vi "Import from VASP DB.vi"(8 "error in (no error)":errorcluster) -> (0 "error out":errorcluster, 3 "All DFT Data Summary":T1)   [LabVIEW 2010]
uses:
  <vilib>/addons/database/Connection.llb/Conn ObjectReference.ctl
  <vilib>/addons/database/_DB Variant To Data/Database Variant To Data.xnode
  <vilib>/addons/database/Connection.llb/DB Tools Open Connec (Path).vi
  <vilib>/addons/database/Connection.llb/Conn Execute.vi
  <vilib>/addons/database/Recordset.llb/Rec Fetch Recordset Data (R).vi
  <vilib>/addons/database/Recordset.llb/Rec Destroy - Connection.vi
  <vilib>/addons/database/NI_Database_API.lvlib
panel:
  in  "Append to Last?":bool
  in  "Pre-Load Raw?":bool
  in  "UDL":path=path "D:/Ab-initio/VASP Calcs/VASP DB.udl"
  out "connection reference":T2
  in  "Cancel":bool
  in  "OK":bool
  in  "Search":bool
  in  "Query Build Cluster":T3={"Sample Check box"=TRUE, "Sample Comparison Type"="Contains", "Sample Name"="", "Logical Sample-Lot "="OR", "LotID Checkbox"=TRUE, "Lot Comparison Type"="Contains", "LotID Name"="", "Logical Lot-Date"="OR", "Date Checkbox"=TRUE, "Start Date"=timestamp(3375812149.928578 s since 1904-01-01), "End Date"=timestamp(3375812149.928578 s since 1904-01-01), "1st search column name"="Folder", "2nd search column name"="Pre_Structure"} {"Start Date" format="%<%X\n%x>T"; "End Date" format="%<%X\n%x>T"}
  in  "DFT Summary":i32(listbox)
  # "Get all results where"
  # "where"
  # "between these dates"
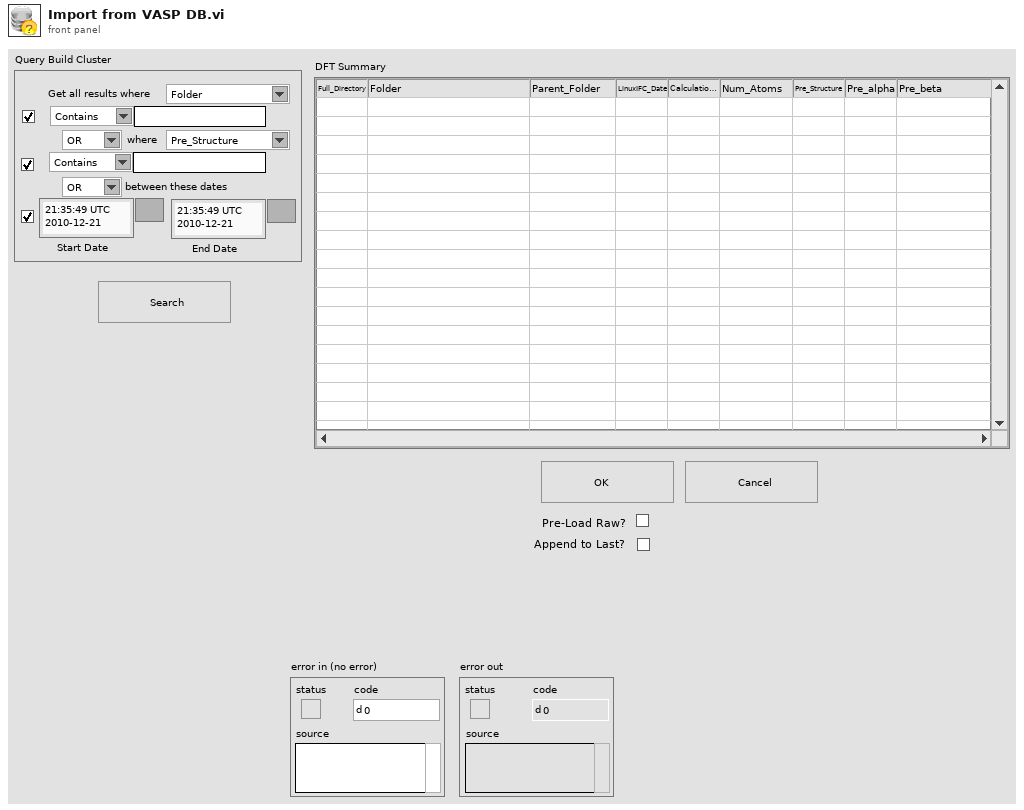
[diagram p1: front panel]
types:
  T1 = cluster{"Headers":string[], "Relaxation Data":string[][]}
  T2 = typedef "NI_Database_API.lvlib/Conn ObjectReference.ctl" = refnum<k1>
  T3 = cluster{"Sample Check box":bool, "Sample Comparison Type":string, "Sample Name":string, "Logical Sample-Lot ":string, "LotID Checkbox":bool, "Lot Comparison Type":string, "LotID Name":string, "Logical Lot-Date":string, "Date Checkbox":bool, "Start Date":timestamp, "End Date":timestamp, "1st search column name":string, "2nd search column name":string}
  T4 = typedef "NI_Database_API.lvlib/Rec ObjectReference.ctl" = refnum<k1>
  T5 = cluster{"ColHdrString":string[], "ItemNames":string[][]}
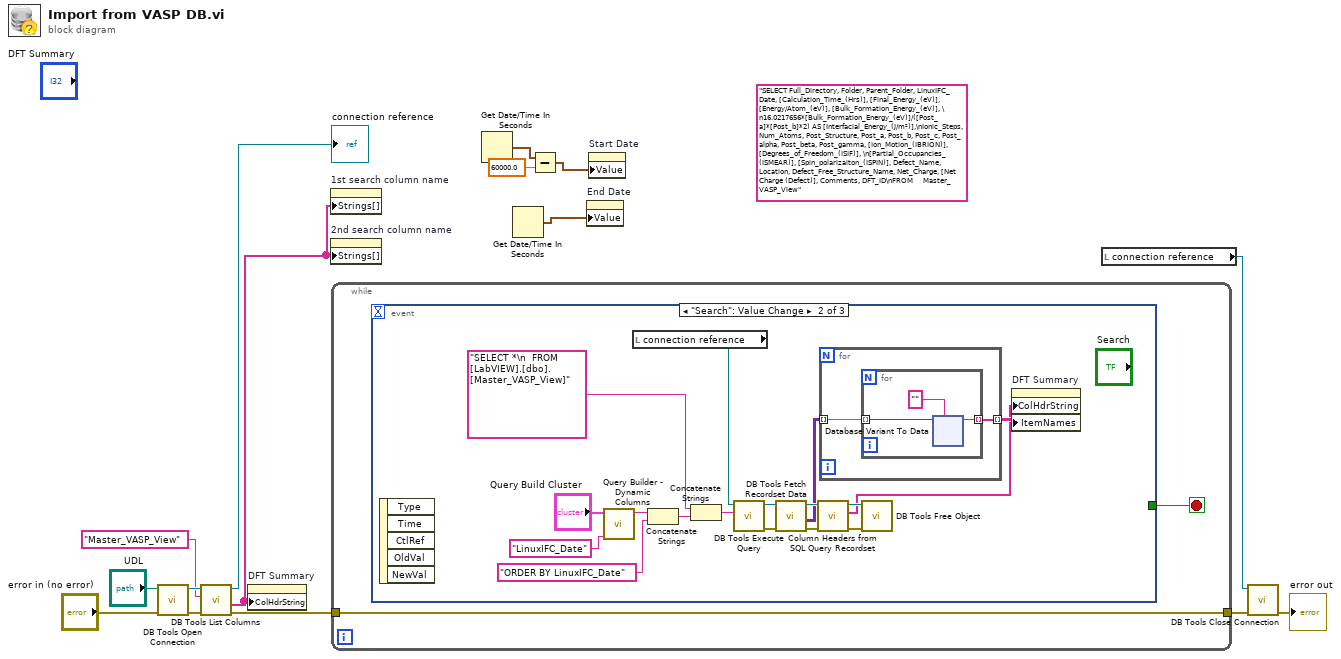
[diagram p0: block diagram]
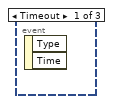
[diagram p2: hidden frame]
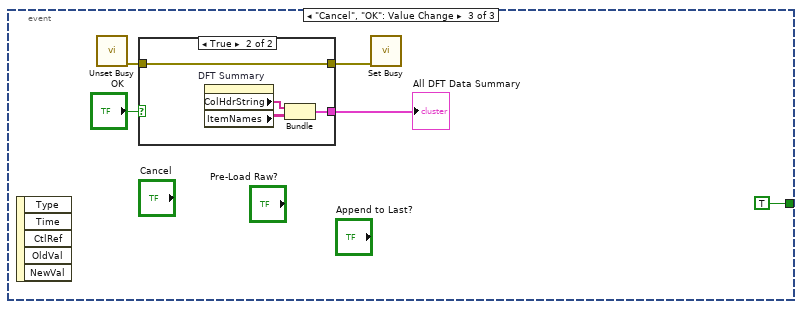
[diagram p3: hidden frame]
diagram:
  (unwired) "SELECT Full_Directory, Folder, Parent_Folder, LinuxIFC_Date, [Calculation_Time_(Hrs)], [Final_Energy_(eV)], [Energy/Atom_(eV)], [Bulk_Formation_Energy_(eV)], \n16.0217656*[Bulk_Formation_Energy_(eV)]/([Post_a]*[Post_b]*2) AS [Interfacial_Energy_(J/m²)],\nIonic_Steps, Num_Atoms, Post_Structure, Post_a, Post_b, Post_c, Post_alpha, Post_beta, Post_gamma, [Ion_Motion_(IBRION)], [Degrees_of_Freedom_(ISIF)], \n[Partial_Occupancies_(ISMEAR)], [Spin_polarizaiton_(ISPIN)], Defect_Name, Location, Defect_Free_Structure_Name, Net_Charge, [Net Charge (Defect)], Comments, DFT_ID\nFROM     Master_VASP_View"
  n1 = call-poly <vilib>:"DB Tools Open Connection.vi"("error in (no error)"="error in (no error)", "connection information"="UDL") -> ("error out"=w9:errorcluster, "connection reference"=w14:T2)  [unwired: 6 in]
  n2 = call <vilib>:"DB Tools List Columns.vi"("error in (no error)"=w9, "table"="Master_VASP_View", "connection reference"=w14) -> ("error out"=w8:errorcluster, "columns"=w11:string[], "connection reference out"=→"connection reference":T2)  [unwired: 1 in, 1 out]
  n3 = property on="DFT Summary" class="MCListbox (strict)"("ColHdrString"=w11) -> ()  [unwired: 2 in, 2 out]
  n4 = property on="1st search column name" class="CmbBox"("Strings[]"=w11) -> ()  [unwired: 2 in, 2 out]
  n5 = property on="2nd search column name" class="CmbBox"("Strings[]"=w11) -> ()  [unwired: 2 in, 2 out]
  n6 = while {
    tunnel: w8 -> [w16]
    tunnel: [w16] -> w5
    stop <- w17 stop-if-true
    n7 = event shown="[1] \"Search\": Value Change" {
      selector: _ -> [_ _ _]
      dyn-events: _ -> [_ _ _]
      timeout: _ -> [_ _ _]
      tunnel: [_ _ TRUE ("Cancel")] -> w17
      event Timeout {
        n8 = event-data() -> ()  [unwired: 1 in, 2 out]
      }
      event "Search": Value Change {
        n9 = event-data() -> ()  [unwired: 1 in, 5 out]
        n10 = call "Query Builder - Dynamic Columns.vi"("Date-Time Column Name"="LinuxIFC_Date", "Query Build Cluster"="Query Build Cluster") -> ("Where Statement"=w30:string)  [unwired: 9 in]
        n11 = local read "connection reference"() -> (w21:T2)
        n12 = Concatenate Strings(w30, "ORDER BY LinuxIFC_Date" ("string")) -> (w18:string)
        n13 = Concatenate Strings("SELECT *\n  FROM [LabVIEW].[dbo].[Master_VASP_View]", w18) -> (w28:string)
        n14 = call-poly <vilib>:"DB Tools Execute Query.vi"("SQL query"=w28, "connection reference"=w21) -> ("error out"=w24:errorcluster, "recordset reference"=w27:T4)  [unwired: 6 in]
        n15 = call-poly <vilib>:"DB Tools Fetch Recordset Data.vi"("error in (no error)"=w24, "recordset reference"=w27) -> ("error out"=w22:errorcluster, "recordset data"=w20:variant[][], "recordset reference out"=w26:T4)  [unwired: 3 in]
        n16 = call "Column Headers from SQL Query Recordset.vi"("error in (no error)"=w22, "recordset reference"=w26) -> ("error out"=w23:errorcluster, "columns"=w19:string[], "Recordset reference Out"=w25:T4)  [unwired: 6 in, 1 out]
        n17 = for {
          tunnel: w20 -> [w36] mode=indexing
          tunnel: [w35] -> w32 mode=indexing
          n18 = for {
            tunnel: w36 -> [w39] mode=indexing
            tunnel: [w37] -> w35 mode=indexing
            n19 = xnode "Database Variant To Data"("database variant"=w39, "type"="") -> ("data"=w37:string)  [unwired: 1 in, 1 out]
          }
        }
        n20 = call-poly <vilib>:"DB Tools Free Object.vi"("error in (no error)"=w23, "recordset reference"=w25) -> ()  [unwired: 8 in, 2 out]
        n21 = property on="DFT Summary" class="MCListbox (strict)"("ColHdrString"=w19, "ItemNames"=w32) -> ()  [unwired: 2 in, 2 out]
      }
      event "Cancel", "OK": Value Change {
        n22 = event-data() -> ()  [unwired: 1 in, 5 out]
        n23 = call <vilib>:"Unset Busy.vi"() -> ("error out"=w73:errorcluster)  [unwired: 11 in]
        n24 = case shown="True" "OK" {
          tunnel: [_ w78] -> w74
          tunnel: w73 -> [_ w77]
          tunnel: [_ w77] -> w72
          frame False {
          }
          frame True {
            n25 = property on="DFT Summary" class="MCListbox (strict)"() -> ("ColHdrString"=w79:string[], "ItemNames"=w80:string[][])  [unwired: 2 in, 2 out]
            n26 = Bundle("ColHdrString"=w79, "ItemNames"=w80) -> (w78:T5)  [unwired: 1 in]
          }
        }
        "All DFT Data Summary" <- w74
        n27 = call <vilib>:"Set Busy.vi"("error in (no error)"=w72) -> ()  [unwired: 9 in, 2 out]
      }
    }
  }
  n28 = Get Date/Time In Seconds() -> (seconds since 1Jan1904=w2:timestamp)
  n29 = Get Date/Time In Seconds() -> (seconds since 1Jan1904=w4:timestamp)
  n30 = Subtract(x=w2, y=60000.0) -> (x-y=w1:timestamp)
  n31 = property on="End Date" class="AbsTime (strict)"("Value"=w4) -> ()  [unwired: 2 in, 2 out]
  n32 = property on="Start Date" class="AbsTime (strict)"("Value"=w1) -> ()  [unwired: 2 in, 2 out]
  n33 = local read "connection reference"() -> (w15:T2)
  n34 = call <vilib>:"DB Tools Close Connection.vi"("error in (no error)"=w5, "connection reference"=w15) -> ("error out"=→"error out":errorcluster)  [unwired: 5 in]
